vi "Read Holding Registers Request.vi"(8 "error in":errorcluster, 9 "Number of Registers":u16, 10 "Starting Address":u16) -> (0 "error out":errorcluster, 2 "modbus data unit out":refnum<class "Modbus Data Unit.lvclass">)   [LabVIEW 2021, in "Master Function Definition.lvclass"]
doc: "This VI forms a modbus data unit for reading multiple holding registers."
uses:
  Master Function Definition.lvclass
  Modbus Data Unit/Modbus Data Unit.lvclass
  Modbus Data Unit/Function.ctl
  Modbus Data Unit/Modbus Data Unit.lvclass/Modbus Data Unit.ctl
  Modbus Data Unit/Construct PDU.vi
  Master Function Definition.lvclass/Master Function Definition.ctl
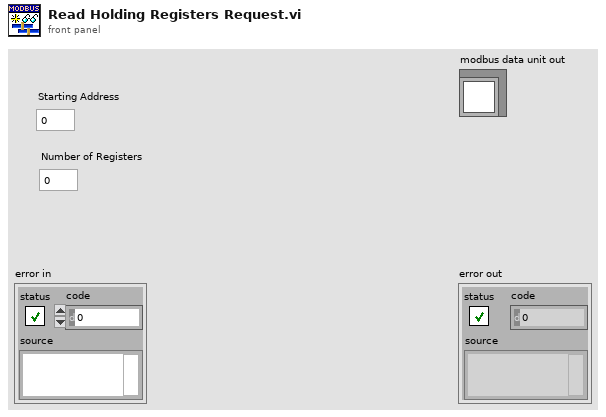
[diagram p1: front panel]
types:
  T1 = typedef "Modbus Data Unit.lvclass/Function.ctl" = u8
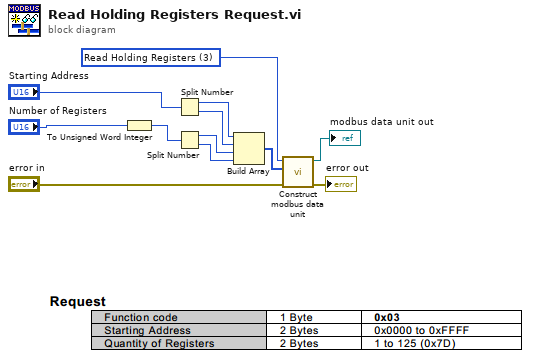
[diagram p0: block diagram]
diagram:
  w3 = T1 3 items=["Read Discrete Inputs"=2, "Read Coils"=1, "Write Single Coil"=5, "Write Multiple Coils"=15, "Read Input Register"=4, "Read Holding Registers"=3, "Write Single Register"=6, "Write Multiple Registers"=16, "Read/Write Multiple Registers"=23, "Mask Write Register"=22, "Read FIFO Queue"=24, "Read File Record"=20, "Write File Record"=21, "Read Exception Status"=7, "Diagnostic"=8, "Get Com Event Counter"=11, "Get Com Event Log"=12, "Report Slave ID"=17, "Read Device Identification"=43] ("Function")
  n1 = To Unsigned Word Integer(number="Number of Registers") -> (unsigned 16bit integer=w2:u16)
  n2 = Split Number(x="Starting Address") -> (hi(x)=w5:u8, lo(x)=w6:u8)
  n3 = Split Number(x=w2) -> (hi(x)=w7:u8, lo(x)=w8:u8)
  n4 = Build Array(w5, w6, w7, w8) -> (w4:u8[])
  n5 = call "Construct modbus data unit.vi"("error in"="error in", "data"=w4, "Function"=w3) -> ("error out"=→"error out":errorcluster, "modbus data unit out"=→"modbus data unit out":refnum<class "Modbus Data Unit.lvclass">)  [unwired: 7 in]
